vi "Read Payload.vi"(8 "error in (no error)":errorcluster, 11 "GodotServer in":refnum<class "GodotServer.lvclass">) -> (0 "error out":errorcluster, 2 "Payload":string, 3 "GodotServer out":refnum<class "GodotServer.lvclass">)   [LabVIEW 2020, in "GodotLV.lvlib" / "GodotServer.lvclass"]
uses:
  GodotServer.lvclass
  <vilib>/IlluminatedG/IG WebSocket Stream/Stream-Websocket/WebsocketStream/WebsocketStream.lvclass
  C:/Program Files (x86)/National Instruments/LabVIEW 2020/vi.lib/IlluminatedG/lv-stream/stream/Stream.lvclass
  GodotServer.lvclass/GodotServer.ctl
  <vilib>/IlluminatedG/lv-stream/stream/Stream.lvclass
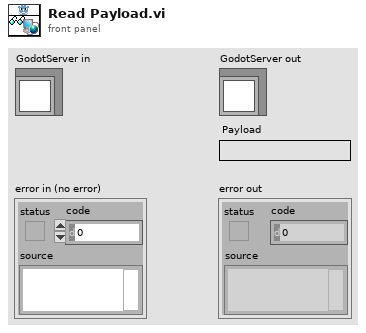
[diagram p1: front panel]
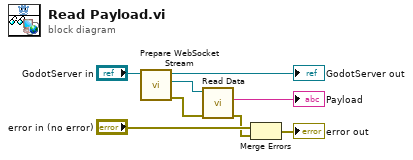
[diagram p0: block diagram]
diagram:
  n1 = call "Prepare WebSocket Stream.vi"("GodotServer in"="GodotServer in") -> ("error out"=w4:errorcluster, "WebsocketStream"=w5:refnum<class "WebsocketStream.lvclass">, "GodotServer out"=→"GodotServer out":refnum<class "GodotServer.lvclass">)  [unwired: 8 in]
  n2 = call <vilib>:"Read Data.vi"("error in (no error)"=w4, "Stream in"=w5) -> ("error out"=w1:errorcluster, "Data"=→"Payload":string)  [unwired: 7 in, 1 out]
  n3 = Merge Errors("error in (no error)", w1) -> (→"error out":errorcluster)
